vi "Adjust PID Gains.vi"(9 "Obstacle detected":bool, 10 "Obst PID":T1={"proportional gain (Kc)"=0.015, "integral time (Ti, min)"=0.0045, "derivative time (Td, min)"=0.0} {"derivative time (Td, min)" format="%.6f"; "integral time (Ti, min)" format="%.6f"; "proportional gain (Kc)" format="%.6f"}, 11 "Std PID":T1={"proportional gain (Kc)"=0.01, "integral time (Ti, min)"=0.003, "derivative time (Td, min)"=0.0} {"derivative time (Td, min)" format="%.6f"; "integral time (Ti, min)" format="%.6f"; "proportional gain (Kc)" format="%.6f"}) -> (3 "PID out":T1={"proportional gain (Kc)"=0.01, "integral time (Ti, min)"=0.003, "derivative time (Td, min)"=0.0} {"derivative time (Td, min)" format="%.6f"; "integral time (Ti, min)" format="%.6f"; "proportional gain (Kc)" format="%.6f"})   [LabVIEW 2017]
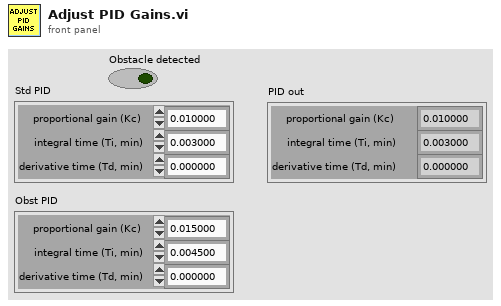
[diagram p1: front panel]
types:
  T1 = cluster{"proportional gain (Kc)":dbl, "integral time (Ti, min)":dbl, "derivative time (Td, min)":dbl}
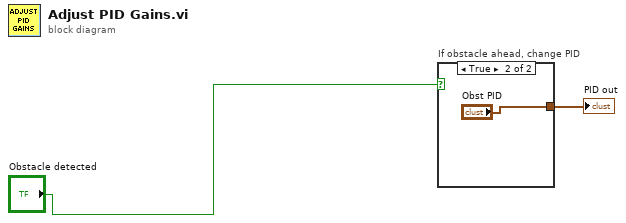
[diagram p0: block diagram]
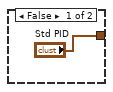
[diagram p2: hidden frame]
diagram:
  n1 = case "If obstacle ahead, change PID" shown="True" "Obstacle detected" {
    tunnel: ["Std PID" "Obst PID"] -> w2
    frame False {
    }
    frame True {
    }
  }
  "PID out" <- w2
